vi "subvi PUMP SWITCH.vi"(11 "error in (no error)":errorcluster) -> (1 "error out":errorcluster, 2 "data out":bool, 3 "data out 2":bool)   [LabVIEW 2016]
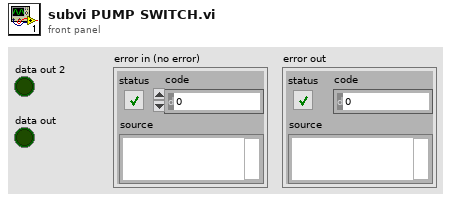
[diagram p1: front panel]
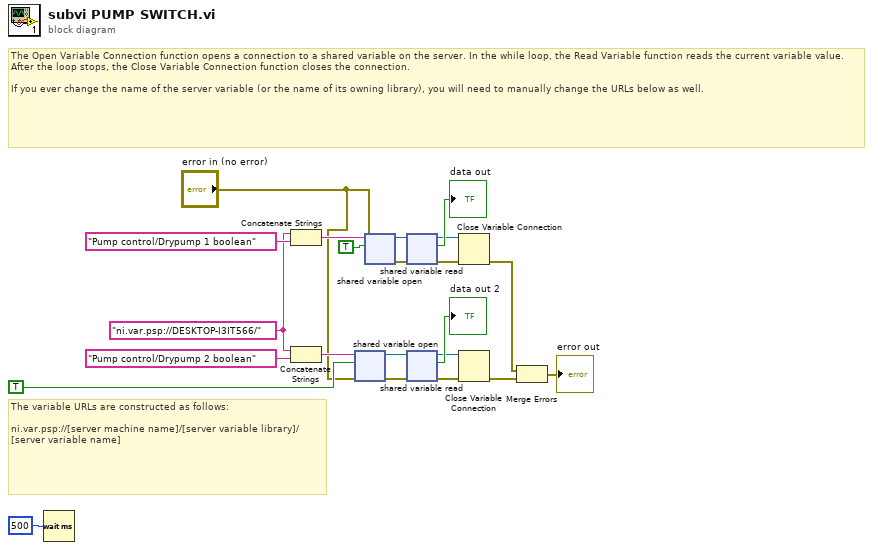
[diagram p0: block diagram]
diagram:
  w3 = "ni.var.psp://DESKTOP-I3IT566/" ("string")
  # "The Open Variable Connection function opens a connection to a shared variable on the server. In the while loop, the Read Variable function reads the current variable value. After the loop stops, the Close Variable Connection function closes the connection.\n\nIf you ever change the name of the server variable (or the name of its owning library), you will need to manually change the URLs below as well."
  # "The variable URLs are constructed as follows:\n\nni.var.psp://[server machine name]/[server variable library]/[server variable name]"
  n1 = Wait (ms)(milliseconds to wait=u32 500 ("millisecond multiple")) -> ()  [unwired: 1 out]
  n2 = Concatenate Strings(w3, "Pump control/Drypump 1 boolean") -> (w17:string)
  n3 = Concatenate Strings(w3, "Pump control/Drypump 2 boolean") -> (w7:string)
  n4 = shared-variable-open(w7, "error in (no error)", TRUE) -> (w11:refnum<k21>, w10:errorcluster)  [unwired: 1 in]
  n5 = shared-variable-open(w17, "error in (no error)", TRUE) -> (w12:refnum<k21>, w13:errorcluster)  [unwired: 1 in]
  n6 = shared-variable-read(w12, w13) -> (w14:refnum<k21>, w16:errorcluster, →"data out":bool)  [unwired: 1 out]
  n7 = shared-variable-read(w11, w10) -> (w9:refnum<k21>, w8:errorcluster, →"data out 2":bool)  [unwired: 1 out]
  n8 = Close Variable Connection(8:w16, 11:w14) -> (0:w15:errorcluster)
  n9 = Close Variable Connection(8:w8, 11:w9) -> (0:w5:errorcluster)
  n10 = Merge Errors(w15, w5) -> (→"error out":errorcluster)
